vi "Simulated Temp.vi"() -> (3 "Simulated Temp":dbl(graph))   [LabVIEW 2017]
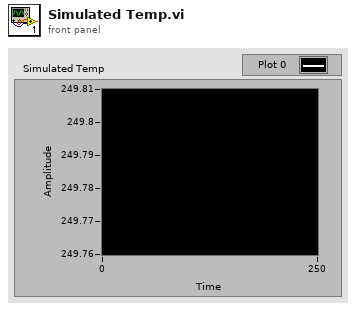
[diagram p1: front panel]
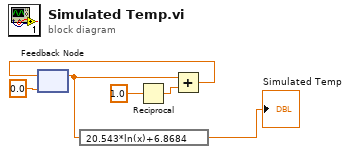
[diagram p0: block diagram]
diagram:
  n1 = feedback #1(0.0) -> (w4:dbl)
  n2 = expression code="20.543*ln(x)+6.8684"(w4) -> (→"Simulated Temp":dbl)
  n3 = Reciprocal(x=1.0) -> (1/x=w3:dbl)
  n4 = Add(x=w4, y=w3) -> (x+y=w6:dbl)
  n5 = feedback-in #1(w6) -> ()
